vi "Measurement UI.vi"() -> ()   [LabVIEW 2024, in "Pure Tone Generation (N Ch) UI.lvlib"]
uses:
  Pure Tone Generation (N Ch) UI.lvlib
  <vilib>/Utility/error.llb/Trim Whitespace One-Sided.vi
panel:
  in  "pure tone configurations":T1(array[cluster])=[{"channel"="Dev1/ao0", "frequency"=997.0, "amplitude"=1.0, "offset"=0.0}, {"channel"="4468_4/ao1", "frequency"=997.0, "amplitude"=1.0, "offset"=0.0}] {"offset" min=-360.0 max=360.0 step=10.0 format="%#_g V"; "amplitude" min=0.0 max=10.0 format="%_4g V"; "frequency" min=0.001 step=10.0 format="%#_4g Hz"}
  in  "offsets":dbl[](array[numeric])
  in  "amplitudes":dbl[](array[numeric])
  in  "frequencies":dbl[](array[numeric])
  in  "physical channels":string[](array[string])
  out "error code out":i32
  out "error description out":string="Empty"
  out "error out":bool
  out "Task":u16(ring)
  out "generator status":string="Idle"
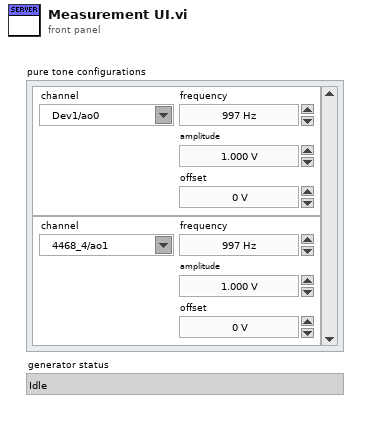
[diagram p1: front panel]
types:
  T1 = cluster{"channel":tag, "frequency":dbl, "amplitude":dbl, "offset":dbl}[]
  T2 = cluster{"channel":tag, "frequency":dbl, "amplitude":dbl, "offset":dbl}
  T3 = enum8{"Enabled", "Disabled", "Disabled and Grayed Out"}
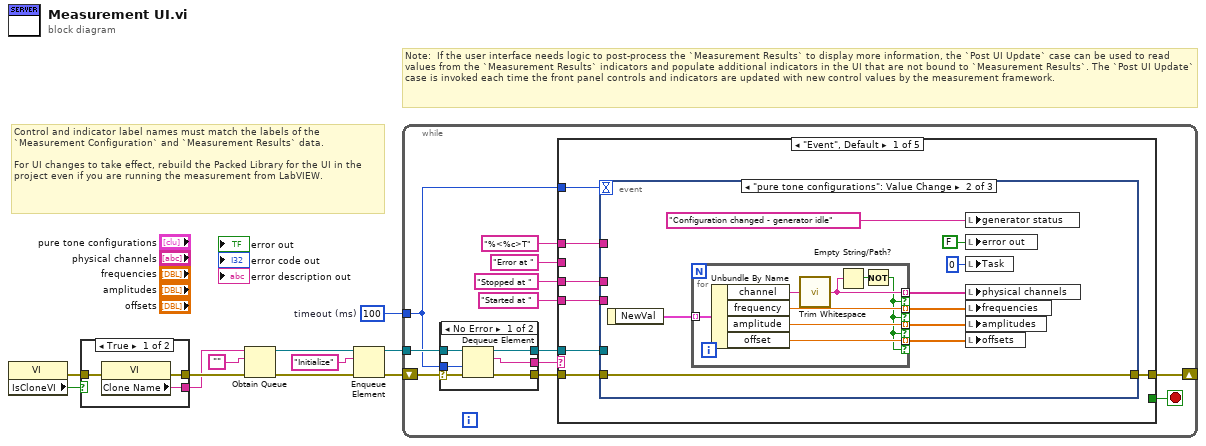
[diagram p0: block diagram]
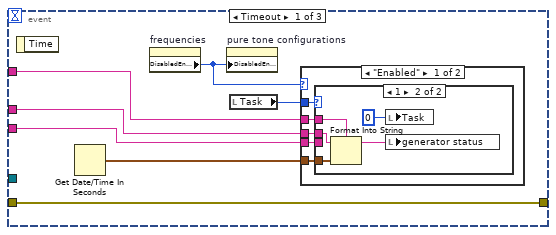
[diagram p2: hidden frame]
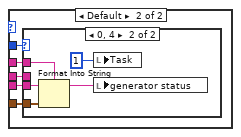
[diagram p4: hidden frame]
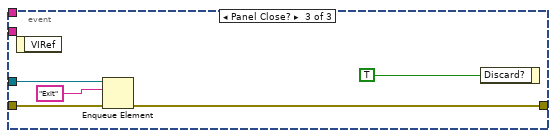
[diagram p6: hidden frame]
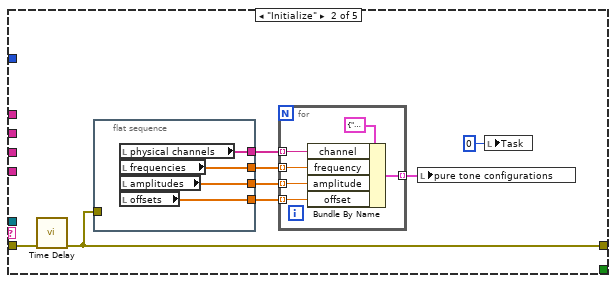
[diagram p7: hidden frame]
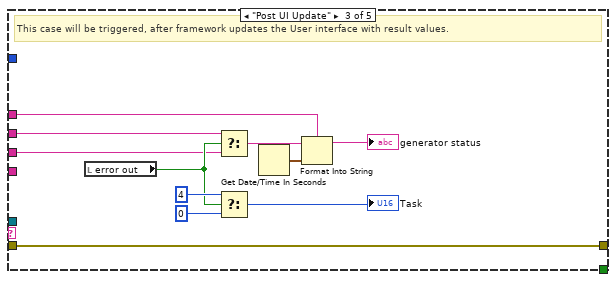
[diagram p8: hidden frame]
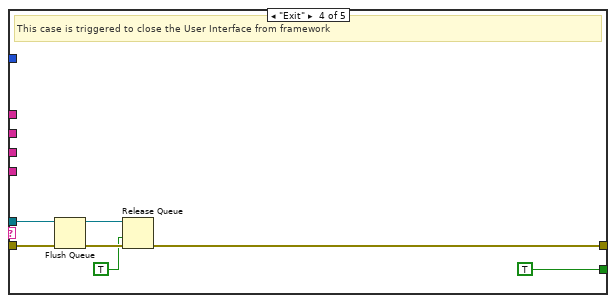
[diagram p9: hidden frame]
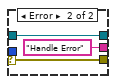
[diagram p11: hidden frame]
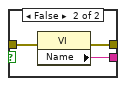
[diagram p12: hidden frame]
diagram:
  w1 = 100  # timeout (ms)
  # "Note:  If the user interface needs logic to post-process the `Measurement Results` to display more information, the `Post UI Update` case can be used to read values from the `Measurement Results` indicators and populate additional indicators in the UI that are not bound to `Measurement Results`. The `Post UI Update` case is invoked each time the front panel controls and indicators are updated with new control values by the measurement framework."
  # "Control and indicator label names must match the labels of the `Measurement Configuration` and `Measurement Results` data. \n\nFor UI changes to take effect, rebuild the Packed Library for the UI in the project even if you are running the measurement from LabVIEW."
  n1 = property class="VI"() -> (error out=w2:errorcluster, "IsCloneVI"=w3:bool)  [unwired: 2 in, 1 out]
  n2 = case shown="True" w3 {
    tunnel: [w14 w17] -> w11
    tunnel: [w13 w16] -> w10
    tunnel: w2 -> [w12 w15]
    frame True {
      n3 = property class="VI"(error in=w12) -> (error out=w14:errorcluster, "Clone Name"=w13:string)  [unwired: 1 in, 1 out]
    }
    frame False {
      n4 = property class="VI"(error in=w15) -> (error out=w17:errorcluster, "Name"=w16:string)  [unwired: 1 in, 1 out]
    }
  }
  n5 = Obtain Queue(name (unnamed)=w10, element data type="", error in (no error)=w11) -> (queue out=w7:refnum<queue>, error out=w9:errorcluster)  [unwired: 2 in, 1 out]
  n6 = Enqueue Element(queue=w7, element="Initialize", error in (no error)=w9) -> (queue out=w6:refnum<queue>, error out=w8:errorcluster)  [unwired: 1 in, 1 out]
  n7 = while {
    shift-right: [w24] -> _
    shift-left: w8 -> [w29]
    tunnel: w6 -> [w27]
    tunnel: w1 -> [w22]
    stop <- w23 stop-if-true
    n8 = case shown="No Error" w29 {
      selector: w29 -> [w128 w131]
      tunnel: [w127 w131] -> w28
      tunnel: w27 -> [w126 w130]
      tunnel: [w125 w130] -> w26
      tunnel: [w124 "Handle Error"] -> w25
      tunnel: w22 -> [w123 _]
      frame No Error {
        n9 = Dequeue Element(queue=w126, timeout in ms (-1)=w123, error in (no error)=w128) -> (queue out=w125:refnum<queue>, element=w124:string, error out=w127:errorcluster)  [unwired: 1 out]
      }
      frame Error {
      }
    }
    n10 = case shown="\"Event\", Default" w25 {
      tunnel: w28 -> [w35 w91 w114 w121 w122]
      tunnel: w26 -> [w34 _ _ w119 _]
      tunnel: [w36 w90 w114 w116 w122] -> w24
      tunnel: [_ _ _ TRUE _] -> w23
      tunnel: w22 -> [w33 _ _ _ _]
      tunnel: "%<%c>T" ("format string") -> [w32 _ w107 _ _]
      tunnel: "Error at " ("current status") -> [_ _ w106 _ _]
      tunnel: "Stopped at " ("current status") -> [w31 _ w105 _ _]
      tunnel: "Started at " ("format string") -> [w30 _ _ _ _]
      frame "Event", Default {
        n11 = event shown="[1] \"pure tone configurations\": Value Change" {
          selector: _ -> [_ _ _]
          dyn-events: _ -> [_ _ _]
          timeout: w33 -> [_ _ _]
          tunnel: [w43 w72 w83] -> w36
          tunnel: w35 -> [w43 w72 w84]
          tunnel: w34 -> [_ _ w82]
          tunnel: w32 -> [w42 _ _]
          tunnel: w31 -> [w41 _ _]
          tunnel: w30 -> [w40 _ _]
          event Timeout {
            n12 = event-data() -> ()  [unwired: 1 in, 1 out]
            n13 = Get Date/Time In Seconds() -> (seconds since 1Jan1904=w39:timestamp)
            n14 = property on="frequencies" class="Arr (strict)"() -> ("DisabledEnum"=w37:T3)  [unwired: 2 in, 2 out]
            n15 = property on="pure tone configurations" class="Arr (strict)"("DisabledEnum"=w37) -> ()  [unwired: 2 in, 2 out]
            n16 = local read "Task"() -> (w38:u16)
            n17 = case shown="\"Enabled\"" w37 {
              tunnel: w38 -> [w48 w58]
              tunnel: w40 -> [w45 w57]
              tunnel: w42 -> [w47 w55]
              tunnel: w39 -> [w46 w56]
              tunnel: w41 -> [w44 w54]
              frame "Enabled" {
                n18 = case shown="1" w48 {
                  tunnel: w47 -> [_ w53]
                  tunnel: w46 -> [_ w52]
                  tunnel: w45 -> [_ _]
                  tunnel: w44 -> [_ w51]
                  frame Default {
                  }
                  frame 1 {
                    n19 = Format Into String(format string=w53, initial string=w51, w52) -> (resulting string=w49:string)  [unwired: 1 in, 1 out]
                    n20 = local write "Task"(u16 0 ("Task")) -> ()
                    n21 = local write "generator status"(w49) -> ()
                  }
                }
              }
              frame Default {
                n22 = case shown="0, 4" w58 {
                  tunnel: w57 -> [_ w63]
                  tunnel: w56 -> [_ w62]
                  tunnel: w55 -> [_ w61]
                  tunnel: w54 -> [_ _]
                  frame Default {
                  }
                  frame 0, 4 {
                    n23 = Format Into String(format string=w61, initial string=w63, w62) -> (resulting string=w59:string)  [unwired: 1 in, 1 out]
                    n24 = local write "Task"(u16 1 ("Task")) -> ()
                    n25 = local write "generator status"(w59) -> ()
                  }
                }
              }
            }
          }
          event "pure tone configurations": Value Change {
            n26 = event-data() -> ("NewVal"=w71:T1)  [unwired: 1 in]
            n27 = for {
              tunnel: w71 -> [w80] mode=indexing
              tunnel: [w78] -> w69 mode=indexing if=w73
              tunnel: [w75] -> w70 mode=indexing if=w73
              tunnel: [w77] -> w68 mode=indexing if=w73
              tunnel: [w76] -> w67 mode=indexing if=w73
              n28 = Unbundle By Name(w80) -> ("channel"=w79:tag, "frequency"=w78:dbl, "amplitude"=w77:dbl, "offset"=w76:dbl)
              n29 = call <vilib>:"Trim Whitespace.vi"("string"=w79) -> ("trimmed string"=w75:string)  [unwired: 1 in]
              n30 = Empty String/Path?(string/path=w75) -> (empty?=w74:bool)
              n31 = Not(x=w74) -> (.not. x?=w73:bool)
            }
            n32 = local write "generator status"("Configuration changed - generator idle" ("current status")) -> ()
            n33 = local write "error out"(FALSE ("error out")) -> ()
            n34 = local write "Task"(u16 0 ("Task")) -> ()
            n35 = local write "physical channels"(w70) -> ()
            n36 = local write "frequencies"(w69) -> ()
            n37 = local write "amplitudes"(w68) -> ()
            n38 = local write "offsets"(w67) -> ()
          }
          event Panel Close? {
            n39 = event-data() -> ()  [unwired: 1 in, 1 out]
            n40 = Enqueue Element(queue=w82, element="Exit", error in (no error)=w84) -> (error out=w83:errorcluster)  [unwired: 1 in, 2 out]
            n41 = event-data("Discard?"=TRUE) -> ()  [unwired: 1 in, 1 out]
          }
        }
      }
      frame "Initialize" {
        n42 = call "Time Delay"("error in (no error)"=w91) -> ("error out"=w90:errorcluster)  [unwired: 10 in]
        n43 = flat-sequence {
          tunnel: w90 -> [_]
          tunnel: [w97] -> w89
          tunnel: [w96] -> w88
          tunnel: [w95] -> w87
          tunnel: [w94] -> w86
          frame #0 {
            n44 = local read "physical channels"() -> (w94:string[])
            n45 = local read "frequencies"() -> (w95:dbl[])
            n46 = local read "amplitudes"() -> (w96:dbl[])
            n47 = local read "offsets"() -> (w97:dbl[])
          }
        }
        n48 = for {
          tunnel: [w102] -> w92 mode=indexing
          tunnel: w89 -> [w101] mode=indexing
          tunnel: w88 -> [w100] mode=indexing
          tunnel: w87 -> [w99] mode=indexing
          tunnel: w86 -> [w98] mode=indexing
          n49 = Bundle By Name(cluster=T2 {"channel"="Dev1/ao0", "frequency"=997.0, "amplitude"=1.0, "offset"=0.0} ("output configuration"), "channel"=w98, "frequency"=w99, "amplitude"=w100, "offset"=w101) -> (w102:T2)
        }
        n50 = local write "pure tone configurations"(w92) -> ()
        n51 = local write "Task"(u16 0 ("Task")) -> ()
      }
      frame "Post UI Update" {
        # "This case will be triggered, after framework updates the User interface with result values."
        n52 = local read "error out"() -> (w109:bool)
        n53 = Select(t=w106, s=w109, f=w105) -> (s? t:f=w113:string)
        n54 = Select(t=u16 4 ("Task"), s=w109, f=u16 0 ("Task")) -> (s? t:f=→"Task":u16)
        n55 = Get Date/Time In Seconds() -> (seconds since 1Jan1904=w112:timestamp)
        n56 = Format Into String(format string=w107, initial string=w113, w112) -> (resulting string=→"generator status":string)  [unwired: 1 in, 1 out]
      }
      frame "Exit" {
        # "This case is triggered to close the User Interface from framework"
        n57 = Flush Queue(queue=w119, error in (no error)=w121) -> (queue out=w118:refnum<queue>, error out=w117:errorcluster)  [unwired: 1 out]
        n58 = Release Queue(queue=w118, force destroy? (F)=TRUE, error in (no error)=w117) -> (error out=w116:errorcluster)  [unwired: 2 out]
      }
      frame "Handle Error" {
      }
    }
  }
